vi "atMonochromator_cancelCallback_command_ChangeSlitWidth.vi"(8 "error in (no error)":errorcluster) -> (0 "error out":errorcluster, 3 "function return":i32)   [LabVIEW 2016, in "SALLV_atMonochromator.lvlib"]
doc: "int atMonochromator_shm_cancelCallback_command_ChangeSlitWidthLV();"
uses:
  SALLV_atMonochromator.lvlib
  SALLV_atMonochromator.so
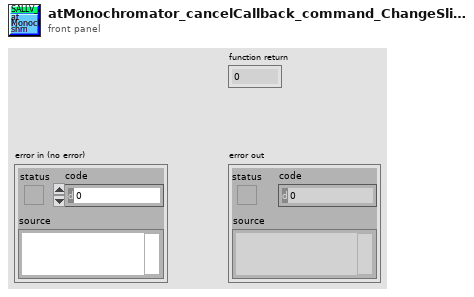
[diagram p1: front panel]
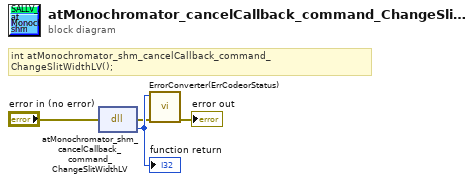
[diagram p0: block diagram]
diagram:
  # "int atMonochromator_shm_cancelCallback_command_ChangeSlitWidthLV();"
  n1 = dll-call lib="home/andres/Desktop/SAL_atMonochromator/SALLV_atMonochromator.*" fn="atMonochromator_shm_cancelCallback_command_ChangeSlitWidthLV"(error in="error in (no error)") -> (error out=w2:errorcluster, w4:i32)  [unwired: 2 in, 1 out]
  "function return" <- w4
  n2 = call "ErrorConverter(ErrCodeorStatus).vi"("error in (no error)"=w2, "error code"=w4) -> ("error out"=→"error out":errorcluster)  [unwired: 9 in]
